vi "Day 16 - Part two.vi"() -> ()   [LabVIEW 2023]
uses:
  <vilib>/Utility/error.llb/Trim Whitespace One-Sided.vi
panel:
  out "loop i":i32
  in  "time left":i32=26
  out "most pressure":i32
  in  "test":bool
  in  "test input":string="Valve AA has flow rate=0; tunnels lead to valves DD, II, BB\nValve BB has flow rate=13; tunnels lead to valves CC, AA\nValve CC has flow rate=2; tunnels lead to valves DD, BB\nValve DD has flow rate=20; tunnels lead to valves CC, AA, EE\nValve EE has flow rate=3; tunnels lead to valves FF, DD\nValve FF has flow rate=0; tunnels lead to valves EE, GG\nValve GG has flow rate=0; tunnels lead to valves FF, HH\nValve HH has flow rate=22; tunnel leads to valve GG\nValve II has flow rate=0; tunnels lead to valves AA, JJ\nValve JJ has flow rate=21; tunnel leads to valve II"
  in  "input":string="Valve DR has flow rate=22; tunnels lead to valves DC, YA\nValve IO has flow rate=14; tunnels lead to valves GE, CK, HY, XB\nValve XY has flow rate=0; tunnels lead to valves IP, AR\nValve UQ has flow rate=0; tunnels lead to valves XU, PD\nValve FO has flow rate=0; tunnels lead to valves DL, NC\nValve PU has flow rate=0; tunnels lead to valves ZJ, AN\nValve MK has flow rate=0; tunnels lead to valves ZS, SB\nValve HN has flow rate=0; tunnels lead to valves AA, DV\nValve XF has flow rate=0; tunnels lead to valves XB, AA\nValve OD has flow rate=13; tunnels lead to valves ZS, AF, SY, QQ, AR\nValve GE has flow rate=0; tunnels lead to valves KR, IO\nValve UF has flow rate=18; tunnels lead to valves QQ, AN, YE, GY\nValve WK has flow rate=19; tunnel leads to valve PQ\nValve PQ has flow rate=0; tunnels lead to valves WK, CW\nValve XU has flow rate=0; tunnels lead to valves DV, UQ\nValve SH has flow rate=0; tunnels lead to valves IP, AA\nValve SY has flow rate=0; tunnels lead to valves ZJ, OD\nValve OU has flow rate=0; tunnels lead to valves CK, DL\nValve IP has flow rate=8; tunnels lead to valves CY, ML, YI, XY, SH\nValve XZ has flow rate=0; tunnels lead to valves AM, PD\nValve ZU has flow rate=0; tunnels lead to valves CW, SB\nValve DC has flow rate=0; tunnels lead to valves CF, DR\nValve QY has flow rate=0; tunnels lead to valves CW, MQ\nValve XB has flow rate=0; tunnels lead to valves IO, XF\nValve AF has flow rate=0; tunnels lead to valves PD, OD\nValve GY has flow rate=0; tunnels lead to valves UF, ZC\nValve ZC has flow rate=0; tunnels lead to valves GY, CW\nValve ZJ has flow rate=25; tunnels lead to valves SY, PU\nValve NC has flow rate=6; tunnels lead to valves HY, ML, NJ, AT, FO\nValve DS has flow rate=0; tunnels lead to valves AT, DV\nValve DV has flow rate=7; tunnels lead to valves FD, KR, HN, DS, XU\nValve HY has flow rate=0; tunnels lead to valves NC, IO\nValve WF has flow rate=0; tunnels lead to valves NJ, AA\nValve CK has flow rate=0; tunnels lead to valves IO, OU\nValve YE has flow rate=0; tunnels lead to valves CY, UF\nValve LA has flow rate=0; tunnels lead to valves DL, ZM\nValve QQ has flow rate=0; tunnels lead to valves OD, UF\nValve AM has flow rate=0; tunnels lead to valves XZ, SB\nValve AN has flow rate=0; tunnels lead to valves UF, PU\nValve CL has flow rate=16; tunnels lead to valves YA, LD\nValve CF has flow rate=12; tunnel leads to valve DC\nValve FD has flow rate=0; tunnels lead to valves DV, DL\nValve QU has flow rate=0; tunnels lead to valves LD, PD\nValve AT has flow rate=0; tunnels lead to valves DS, NC\nValve SB has flow rate=24; tunnels lead to valves MK, AM, ZU\nValve YI has flow rate=0; tunnels lead to valves DL, IP\nValve ZM has flow rate=0; tunnels lead to valves AA, LA\nValve LD has flow rate=0; tunnels lead to valves CL, QU\nValve AR has flow rate=0; tunnels lead to valves OD, XY\nValve DL has flow rate=5; tunnels lead to valves FO, LA, YI, OU, FD\nValve MQ has flow rate=0; tunnels lead to valves QY, PD\nValve PD has flow rate=9; tunnels lead to valves MQ, QU, XZ, AF, UQ\nValve KR has flow rate=0; tunnels lead to valves GE, DV\nValve CY has flow rate=0; tunnels lead to valves YE, IP\nValve AA has flow rate=0; tunnels lead to valves SH, XF, ZM, HN, WF\nValve NJ has flow rate=0; tunnels lead to valves NC, WF\nValve YA has flow rate=0; tunnels lead to valves CL, DR\nValve ML has flow rate=0; tunnels lead to valves NC, IP\nValve CW has flow rate=15; tunnels lead to valves QY, PQ, ZC, ZU\nValve ZS has flow rate=0; tunnels lead to valves MK, OD\n"
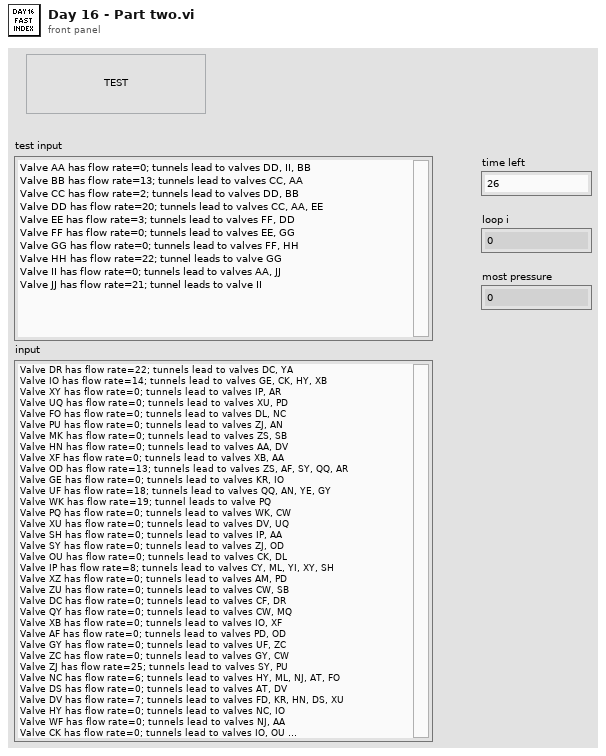
[diagram p1: front panel]
types:
  T1 = cluster{"bitfield":u32, "time left":i32, "index":i32}
  T2 = cluster{"distance[]":cluster{"index":i32, "distance":i32}[], "index":i32}
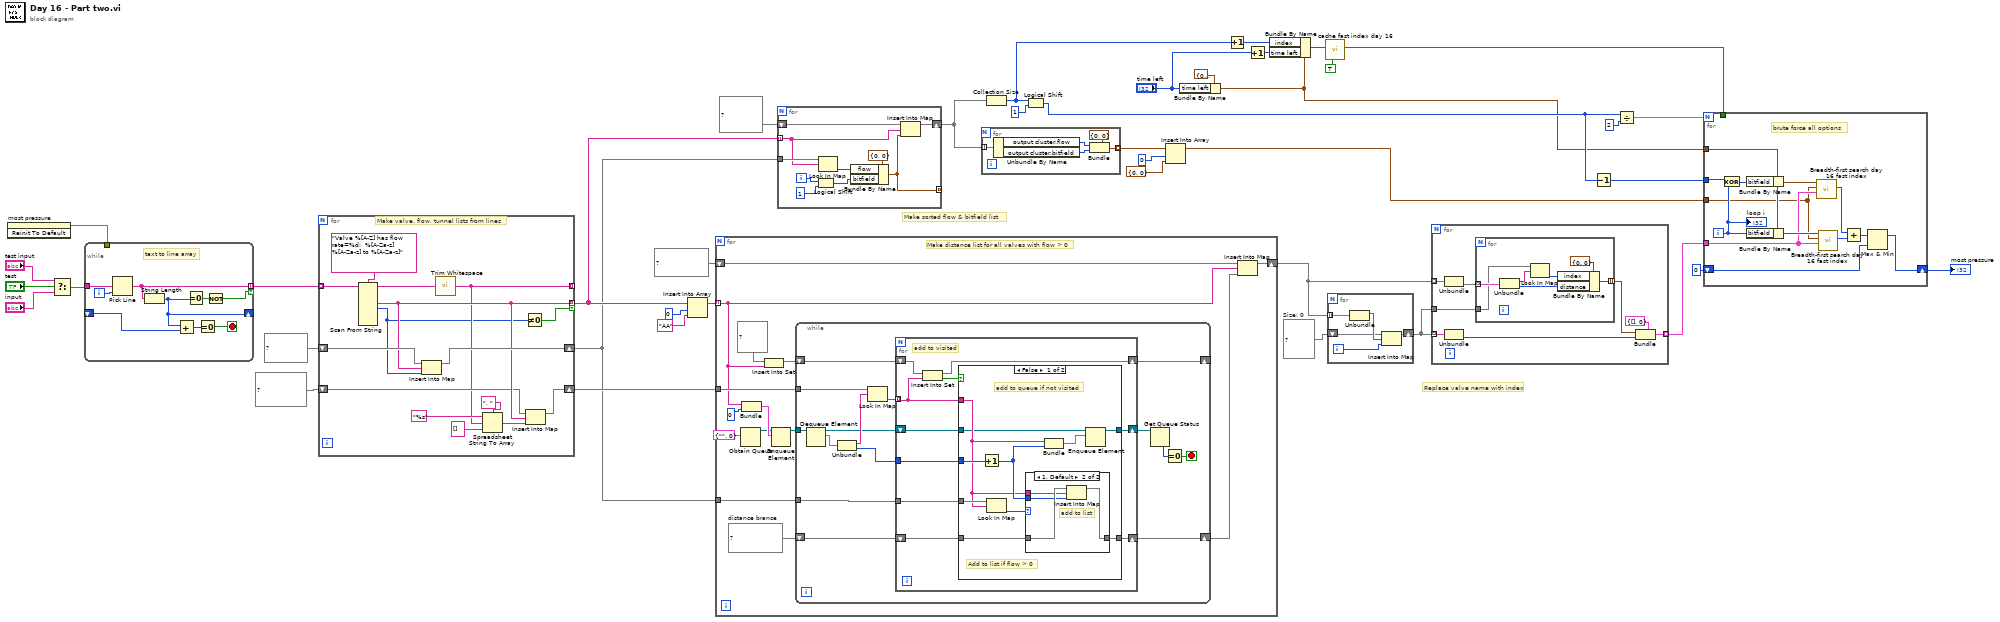
[diagram p0: block diagram]
diagram:
  w21 = map{string, i32} {}  # Size: 0
  # "Replace valve name with index"
  # "Make sorted flow & bitfield list"
  n1 = invoke on="most pressure" class="DigNum (strict)" method="Reinit To Default"() -> (error out=w2:errorcluster)  [unwired: 3 in, 2 out]
  n2 = Select(t="test input", s="test", f="input") -> (s? t:f=w38:string)
  n3 = while {
    tunnel: w38 -> [w49]
    tunnel: [w42] -> w39 mode=indexing if=w48
    shift-right: [w45] -> _
    shift-left: _ -> [w46]
    tunnel: w2 -> [_]
    i -> [w50]
    stop <- w43 stop-if-true
    # "text to line array"
    n4 = Pick Line(multi-line string=w49, line index=w50) -> (output string=w42:string)  [unwired: 1 in]
    n5 = String Length(string=w42) -> (length=w45:i32)
    n6 = Add(x=w45, y=w46) -> (x+y=w47:i32)
    n7 = Equal To 0?(x=w45) -> (x = 0?=w44:bool)
    n8 = Equal To 0?(x=w47) -> (x = 0?=w43:bool)
    n9 = Not(x=w44) -> (.not. x?=w48:bool)
  }
  n10 = for {
    tunnel: w39 -> [w65] mode=indexing
    tunnel: [w61] -> w27 mode=indexing if=w52
    tunnel: [w53] -> _ mode=indexing
    shift-right: [w63] -> w26
    shift-left: map{string, i32} {} ("Size: 0") -> [w62]
    shift-right: [w56] -> w31
    shift-left: map{string, string[]} {} ("Size: 0") -> [w55]
    # "Make valve, flow, tunnel lists from lines"
    n11 = Scan From String(format string="Valve %[A-Z] has flow rate=%d;  %[A-Za-z] %[A-Za-z] to %[A-Za-z]", input string=w65) -> (remaining string=w58:string, output 1=w61:string, output 2=w51:i32)  [unwired: 10 in, 2 out]
    n12 = Insert Into Map(map in=w62, key=w61, value=w51) -> (map out=w63:map{string, i32})  [unwired: 2 out]
    n13 = call <vilib>:"Trim Whitespace.vi"("string"=w58) -> ("trimmed string"=w53:string)  [unwired: 1 in]
    n14 = Spreadsheet String To Array(delimiter (Tab)=", ", format string="%s", spreadsheet string=w53, array type (2D Dbl)=string[] [] ("appended array")) -> (array=w60:string[])
    n15 = Not Equal To 0?(x=w51) -> (x != 0?=w52:bool)
    n16 = Insert Into Map(map in=w55, key=w61, value=w60) -> (map out=w56:map{string, string[]})  [unwired: 2 out]
  }
  n17 = Insert Into Array(array=w27, index=0, new element="AA" ("new element/subarray")) -> (w32:string[])
  n18 = for {
    tunnel: w31 -> [w77]
    tunnel: w26 -> [w78]
    tunnel: w32 -> [w72] mode=indexing
    shift-right: [w74] -> w22
    shift-left: map{string, map{string, i32}} {} ("Size: 0") -> [w75]
    w68 = map{string, i32} {}  # distance brance
    # "Make distance list for all valves with flow > 0"
    n19 = Obtain Queue(element data type=cluster{string, i32} {"", 0} ("output cluster")) -> (queue out=w66:refnum<queue>)  [unwired: 4 in, 2 out]
    n20 = Bundle(w72, "x+1"=0) -> (w70:cluster{string, "x+1":i32})  [unwired: 1 in]
    n21 = Insert Into Set(10:w72, 11:set{string} {} ("Size: 0")) -> (3:w79:set{string})  [unwired: 1 out]
    n22 = Enqueue Element(queue=w66, element=w70) -> (queue out=w73:refnum<queue>)  [unwired: 2 in, 2 out]
    n23 = while {
      tunnel: w78 -> [w92]
      shift-right: [w93] -> _
      shift-left: w79 -> [w94]
      shift-right: [w91] -> w76
      shift-left: w68 -> [w90]
      tunnel: w77 -> [w89]
      tunnel: w73 -> [w87]
      stop <- w81 stop-if-true
      n24 = Dequeue Element(queue=w87) -> (queue out=w83:refnum<queue>, element=w86:cluster{string, i32})  [unwired: 2 in, 2 out]
      n25 = Unbundle(w86) -> (w85:string, w84:i32)
      n26 = Look In Map(map=w89, key=w85) -> (value=w88:string[])  [unwired: 1 in, 1 out]
      n27 = for {
        tunnel: w88 -> [w99] mode=indexing
        shift-right: [w103] -> w93
        shift-left: w94 -> [w104]
        tunnel: w92 -> [w101]
        tunnel: w84 -> [w100]
        shift-right: [w98] -> w91
        shift-left: w90 -> [w97]
        shift-right: [w95] -> w82
        shift-left: w83 -> [w96]
        # "add to visited"
        n28 = Insert Into Set(10:w99, 11:w104) -> (2:w102:bool, 3:w103:set{string})
        n29 = case shown="False" w102 {
          tunnel: w101 -> [w114 _]
          tunnel: w100 -> [w110 _]
          tunnel: w99 -> [w108 _]
          tunnel: [w112 w121] -> w98
          tunnel: w97 -> [w111 w121]
          tunnel: w96 -> [w107 w120]
          tunnel: [w105 w120] -> w95
          frame False {
            # "Add to list if flow > 0"
            # "add to queue if not visited"
            n30 = Increment(x=w110) -> (x+1=w109:i32)
            n31 = Look In Map(map=w114, key=w108) -> (value=w113:i32)  [unwired: 1 in, 1 out]
            n32 = case shown="1, Default" w113 {
              tunnel: w108 -> [_ w116]
              tunnel: [w115 w118] -> w112
              tunnel: w111 -> [w115 w119]
              tunnel: w109 -> [_ w117]
              frame 0 {
              }
              frame 1, Default {
                # "add to list"
                n33 = Insert Into Map(map in=w119, key=w116, value=w117) -> (map out=w118:map{string, i32})  [unwired: 2 out]
              }
            }
            n34 = Bundle(w108, w109) -> (w106:cluster{string, i32})  [unwired: 1 in]
            n35 = Enqueue Element(queue=w107, element=w106) -> (queue out=w105:refnum<queue>)  [unwired: 2 in, 2 out]
          }
          frame True {
          }
        }
      }
      n36 = Get Queue Status(queue=w82) -> (# elements in queue=w80:i32)  [unwired: 2 in, 7 out]
      n37 = Equal To 0?(x=w80) -> (x = 0?=w81:bool)
    }
    n38 = Insert Into Map(map in=w75, key=w72, value=w76) -> (map out=w74:map{string, map{string, i32}})  [unwired: 2 out]
  }
  n39 = for {
    tunnel: w27 -> [w123] mode=indexing
    tunnel: w26 -> [w127]
    shift-right: [w125] -> w11
    shift-left: map{string, cluster{"flow":i32, "bitfield":u32}} {} ("Size: 0") -> [w124]
    tunnel: [w122] -> _ mode=indexing
    i -> [w130]
    n40 = Logical Shift(y=w130, x=u32 1) -> (x << y=w128:u32)
    n41 = Look In Map(map=w127, key=w123) -> (value=w129:i32)  [unwired: 1 in, 1 out]
    n42 = Bundle By Name(cluster=cluster{"flow":i32, "bitfield":u32} {"flow"=0, "bitfield"=0} ("output cluster"), "flow"=w129, "bitfield"=w128) -> (w122:cluster{"flow":i32, "bitfield":u32})
    n43 = Insert Into Map(map in=w124, key=w123, value=w122) -> (map out=w125:map{string, cluster{"flow":i32, "bitfield":u32}})  [unwired: 2 out]
  }
  n44 = for {
    tunnel: w11 -> [w136] mode=indexing
    tunnel: [w133] -> w15 mode=indexing
    n45 = Unbundle By Name(w136) -> ("output cluster.flow"=w135:i32, "output cluster.bitfield"=w134:u32)
    n46 = Bundle(cluster=cluster{"flow":i32, "bitfield":u32} {"flow"=0, "bitfield"=0}, "flow"=w135, "bitfield"=w134) -> (w133:cluster{"flow":i32, "bitfield":u32})
  }
  n47 = Collection Size(1:w11) -> (0:w8:i32)
  n48 = Logical Shift(y=w8, x=u32 1) -> (x << y=w12:u32)
  n49 = Insert Into Array(array=w15, index=0, new element=cluster{"flow":i32, "bitfield":u32} {"flow"=0, "bitfield"=0} ("output cluster")) -> (w18:cluster{"flow":i32, "bitfield":u32}[])
  n50 = Bundle By Name(cluster=T1 {"bitfield"=0, "time left"=0, "index"=0} ("input \n[index, bitfield, time left]"), "time left"="time left") -> (w9:T1)
  n51 = Increment(x=w8) -> (x+1=w4:i32)
  n52 = Increment(x="time left") -> (x+1=w3:i32)
  n53 = Bundle By Name(cluster=w9, "index"=w4, "time left"=w3) -> (w5:T1)
  n54 = call "cache fast index day 16.vi"("Clear"=TRUE, "input \n[index, \nbitfield, \ntime left]"=w5) -> ("key not found?"=w28:bool)  [unwired: 8 in, 1 out]
  n55 = for {
    tunnel: w22 -> [w141] mode=indexing
    shift-right: [w138] -> w20
    shift-left: w21 -> [w137]
    i -> [w139]
    n56 = Unbundle(w141) -> (w140:string)  [unwired: 1 out]
    n57 = Insert Into Map(map in=w137, key=w140, value=w139) -> (map out=w138:map{string, i32})  [unwired: 2 out]
  }
  n58 = for {
    tunnel: w22 -> [w149] mode=indexing
    tunnel: w20 -> [w147] mode=indexing
    tunnel: [w145] -> w19 mode=indexing
    tunnel: w20 -> [w143]
    n59 = Unbundle(w149) -> (w148:map{string, i32})  [unwired: 1 out]
    n60 = Unbundle(w147) -> (w146:i32)  [unwired: 1 out]
    n61 = for {
      tunnel: w148 -> [w156] mode=indexing
      tunnel: [w153] -> w142 mode=indexing
      tunnel: w143 -> [w151]
      n62 = Unbundle(w156) -> ("valve"=w152:string, "distance"=w155:i32)
      n63 = Look In Map(map=w151, key=w152) -> (value=w150:i32)  [unwired: 1 in, 1 out]
      n64 = Bundle By Name(cluster=cluster{"index":i32, "distance":i32} {"index"=0, "distance"=0} ("output cluster"), "index"=w150, "distance"=w155) -> (w153:cluster{"index":i32, "distance":i32})
    }
    n65 = Bundle(cluster=T2 {"distance[]"=[], "index"=0} ("output cluster"), "distance[]"=w142, "index"=w146) -> (w145:T2)
  }
  n66 = Decrement(x=w12) -> (x-1=w10:u32)
  n67 = Divide(x=w12, y=u32 2) -> (x/y=w13:dbl)
  n68 = for {
    N: w13 -> [_]
    tunnel: w9 -> [w165]
    tunnel: w10 -> [w167]
    shift-right: [w161] -> w29
    shift-left: 0 -> [w160]
    tunnel: w28 -> [_]
    tunnel: w19 -> [w158]
    tunnel: w18 -> [w157]
    i -> [w159]
    # "brute force all options"
    n69 = Exclusive Or(1:w159, 2:w167) -> (0:w166:u32)
    n70 = Bundle By Name(cluster=w165, "bitfield"=w166) -> (w168:T1)
    n71 = Bundle By Name(cluster=w165, "bitfield"=w159) -> (w164:T1)
    n72 = call "Breadth-first search day 16 fast index.vi"("distance graph"=w158, "Flow, bitfield"=w157, "input \n[index, bitfield, time left]"=w168) -> ("most pressure"=w169:i32)  [unwired: 8 in]
    n73 = call "Breadth-first search day 16 fast index.vi"("distance graph"=w158, "Flow, bitfield"=w157, "input \n[index, bitfield, time left]"=w164) -> ("most pressure"=w162:i32)  [unwired: 8 in]
    n74 = Add(x=w169, y=w162) -> (x+y=w163:i32)
    n75 = Max & Min(x=w163, y=w160) -> (max(x,y)=w161:i32)  [unwired: 1 out]
    "loop i" <- w159
  }
  "most pressure" <- w29
